vi "Wire Measurement Wrapper.vi"(0 "vi reference":refnum<vi>, 5 "sub vi in":refnum<vi>[](array[refnum]), 7 "terminal":refnum<vi>, 11 "error in":errorcluster) -> (15 "error out":errorcluster)   [LabVIEW 2021, in "Converter.lvlib"]
uses:
  Converter.lvlib
  Converter Reusables/Converter Reusables.lvlib
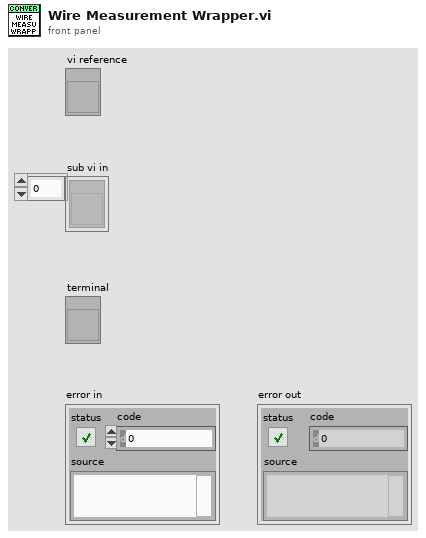
[diagram p1: front panel]
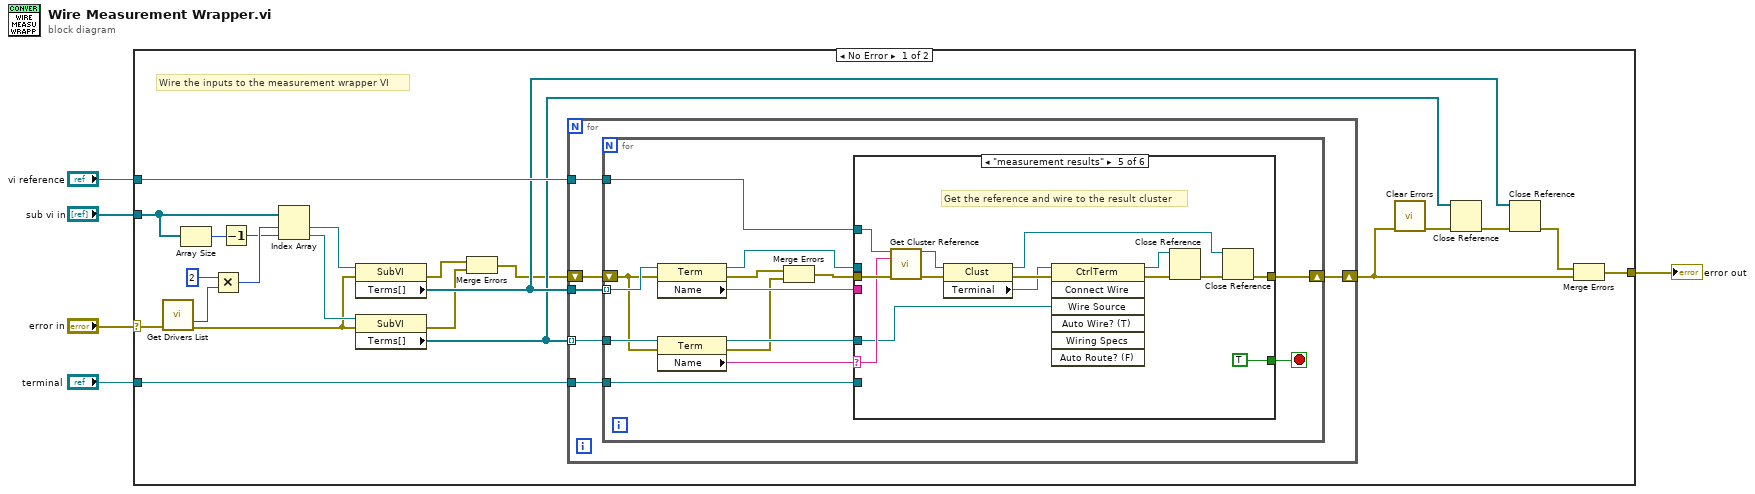
[diagram p0: block diagram]
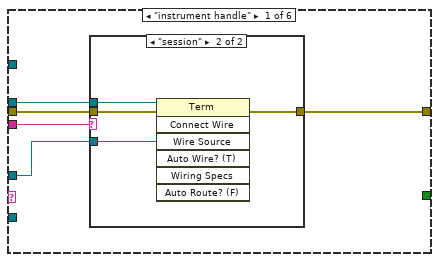
[diagram p2: hidden frame]
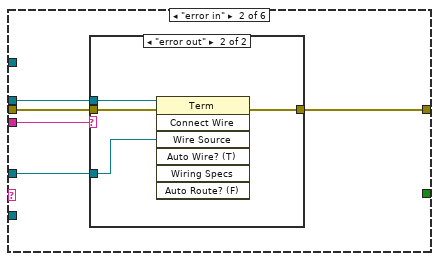
[diagram p4: hidden frame]
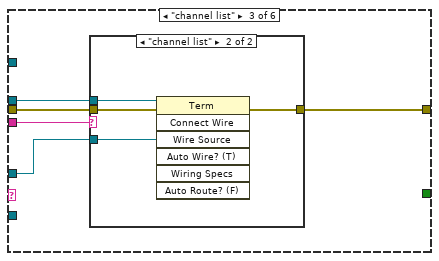
[diagram p6: hidden frame]
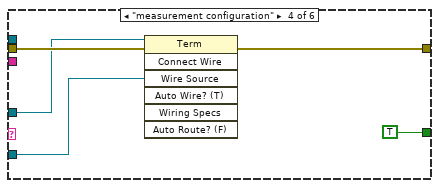
[diagram p8: hidden frame]
diagram:
  n1 = case shown="No Error" "error in" {
    selector: "error in" -> [w15 w98]
    tunnel: "vi reference" -> [w23 _]
    tunnel: [w18 w98] -> w4
    tunnel: "terminal" -> [w16 _]
    tunnel: "sub vi in" -> [w6 _]
    frame No Error {
      # "Wire the inputs to the measurement wrapper VI"
      n2 = call "Get Drivers List.vi"("error in"=w15) -> ("removed duplicates size"=w7:i32, "error out"=w14:errorcluster)  [unwired: 9 in, 4 out]
      n3 = Array Size(array=w6) -> (size(s)=w13:i32)
      n4 = Multiply(x=2, y=w7) -> (x*y=w10:i32)
      n5 = Decrement(x=w13) -> (x-1=w9:i32)
      n6 = Index Array(array=w6, index #1=w10, index #2=w9) -> (element #1=w27:refnum<vi>, element #2=w26:refnum<vi>)
      n7 = property class="SubVI"(reference=w27, error in=w14) -> (error out=w25:errorcluster, "Terms[]"=w22:refnum<vi>[])  [unwired: 1 out]
      n8 = property class="SubVI"(reference=w26, error in=w14) -> (error out=w11:errorcluster, "Terms[]"=w21:refnum<vi>[])  [unwired: 1 out]
      n9 = Merge Errors(w25, w11) -> (w12:errorcluster)
      n10 = for {
        tunnel: w21 -> [w32] mode=indexing
        tunnel: w22 -> [w33]
        tunnel: w16 -> [w31]
        tunnel: w23 -> [w30]
        shift-right: [w29] -> w24
        shift-left: w12 -> [w28]
        n11 = for {
          tunnel: w33 -> [w47] mode=indexing
          tunnel: w32 -> [w46]
          tunnel: w31 -> [w43]
          tunnel: w30 -> [w39]
          shift-right: [w41] -> w29
          shift-left: w28 -> [w37]
          stop <- w38 stop-if-true
          n12 = property class="Term"(reference=w47, error in=w37) -> (reference out=w34:refnum<vi>, error out=w42:errorcluster, "Name"=w40:string)
          n13 = property class="Term"(reference=w46, error in=w37) -> (reference out=w44:refnum<vi>, error out=w35:errorcluster, "Name"=w45:string)
          n14 = Merge Errors(w42, w35) -> (w36:errorcluster)
          n15 = case shown="\"measurement results\"" w45 {
            selector: w45 -> [_ _ _ _ w89 _]
            tunnel: w44 -> [w50 w60 w68 w80 w86 _]
            tunnel: w43 -> [_ _ _ w79 _ _]
            tunnel: w36 -> [w51 w61 w71 w81 w96 w97]
            tunnel: [w48 w58 w69 w82 w91 w97] -> w41
            tunnel: w40 -> [w52 w62 w72 _ _ _]
            tunnel: w34 -> [w49 w59 w70 _ _ _]
            tunnel: w39 -> [_ _ _ _ w90 _]
            tunnel: [_ _ _ TRUE TRUE _] -> w38
            frame "instrument handle" {
              n16 = case shown="\"session\"" w52 {
                tunnel: w51 -> [w53 w57]
                tunnel: w50 -> [_ w54]
                tunnel: w49 -> [_ w56]
                tunnel: [w53 w55] -> w48
                frame Default {
                }
                frame "session" {
                  n17 = invoke class="Term" method="Connect Wire"(reference=w56, error in=w57, "Wire Source"=w54) -> (error out=w55:errorcluster)  [unwired: 4 in, 6 out]
                }
              }
            }
            frame "error in" {
              n18 = case shown="\"error out\"" w62 {
                tunnel: w61 -> [w63 w67]
                tunnel: w60 -> [_ w64]
                tunnel: w59 -> [_ w66]
                tunnel: [w63 w65] -> w58
                frame Default {
                }
                frame "error out" {
                  n19 = invoke class="Term" method="Connect Wire"(reference=w66, error in=w67, "Wire Source"=w64) -> (error out=w65:errorcluster)  [unwired: 4 in, 6 out]
                }
              }
            }
            frame "channel list" {
              n20 = case shown="\"channel list\"" w72 {
                tunnel: w71 -> [w73 w77]
                tunnel: w68 -> [_ w76]
                tunnel: w70 -> [_ w75]
                tunnel: [w73 w74] -> w69
                frame Default {
                }
                frame "channel list" {
                  n21 = invoke class="Term" method="Connect Wire"(reference=w75, error in=w77, "Wire Source"=w76) -> (error out=w74:errorcluster)  [unwired: 4 in, 6 out]
                }
              }
            }
            frame "measurement configuration" {
              n22 = invoke class="Term" method="Connect Wire"(reference=w80, error in=w81, "Wire Source"=w79) -> (error out=w82:errorcluster)  [unwired: 4 in, 6 out]
            }
            frame "measurement results" {
              # "Get the reference and wire to the result cluster"
              n23 = call "Get Cluster Reference.vi"("vi in"=w90, "name/order"=w89, "error in"=w96) -> ("cluster out"=w88:refnum<vi>, "error out"=w95:errorcluster)  [unwired: 11 in]
              n24 = property class="Clust"(reference=w88, error in=w95) -> (reference out=w85:refnum<vi>, error out=w94:errorcluster, "Terminal"=w87:refnum<vi>)
              n25 = invoke class="CtrlTerm" method="Connect Wire"(reference=w87, error in=w94, "Wire Source"=w86) -> (reference out=w84:refnum<vi>, error out=w93:errorcluster)  [unwired: 4 in, 5 out]
              n26 = Close Reference(reference=w84, error in (no error)=w93) -> (error out=w92:errorcluster)
              n27 = Close Reference(reference=w85, error in (no error)=w92) -> (error out=w91:errorcluster)
            }
            frame Default {
            }
          }
        }
      }
      n28 = call <vilib>:"Clear Errors.vi"("error in (no error)"=w24) -> ("error out"=w20:errorcluster)  [unwired: 5 in, 1 out]
      n29 = Close Reference(reference=w21, error in (no error)=w20) -> (error out=w19:errorcluster)
      n30 = Close Reference(reference=w22, error in (no error)=w19) -> (error out=w17:errorcluster)
      n31 = Merge Errors(w17, w24) -> (w18:errorcluster)
    }
    frame Error {
    }
  }
  "error out" <- w4
